vi "GetWSNames.vi"(8 "error in (no error)":errorcluster, 11 "Config":T1) -> (0 "error out":errorcluster, 3 "Names":string[](array[string]))   [LabVIEW 2020]
uses:
  <vilib>/WebServerConfig/Config.ctl
  <vilib>/WebServerConfig/Server.ctl
  <vilib>/WebServerConfig/Alias.ctl
  <vilib>/WebServerConfig/ErrorDocument.ctl
  <vilib>/WebServerConfig/Action.ctl
  <vilib>/WebServerConfig/Redirect.ctl
  <vilib>/WebServerConfig/Interface.ctl
  <vilib>/WebServerConfig/AddHandler.ctl
  <vilib>/WebServerConfig/SSL.ctl
  <vilib>/WebServerConfig/CustomLog.ctl
  <vilib>/WebServerConfig/LoadModule.ctl
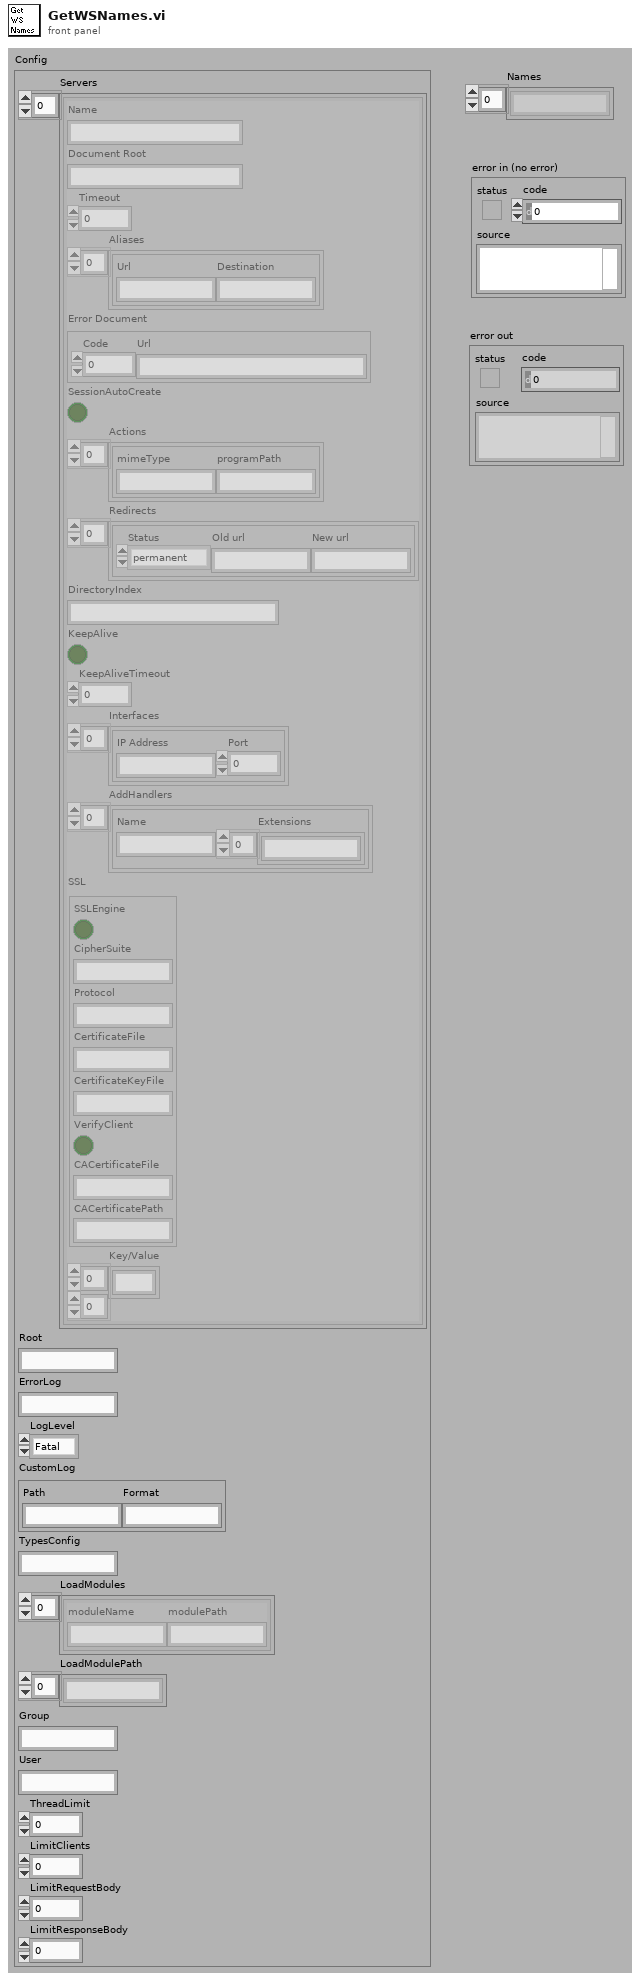
[diagram p1: front panel]
types:
  T1 = typedef "Config.ctl" = cluster{"Servers":T2[], "Root":string, "ErrorLog":string, "LogLevel":enum16{"Fatal", "Error", "Warn", "Info", "Debug", "5", "6", "7", "8", "Verbose"}, "CustomLog":T10, "TypesConfig":string, "LoadModules":T11[], "LoadModulePath":string[], "Group":string, "User":string, "ThreadLimit":u32, "LimitClients":u32, "LimitRequestBody":u32, "LimitResponseBody":u32}
  T2 = typedef "Server.ctl" = cluster{"Name":string, "Document Root":string, "Timeout":u32, "Aliases":T3[], "Error Document":T4, "SessionAutoCreate":bool, "Actions":T5[], "Redirects":T6[], "DirectoryIndex":string, "KeepAlive":bool, "KeepAliveTimeout":u32, "Interfaces":T7[], "AddHandlers":T8[], "SSL":T9, "Key/Value":string[][]}
  T3 = typedef "Alias.ctl" = cluster{"Url":string, "Destination":string}
  T4 = typedef "ErrorDocument.ctl" = cluster{"Code":u16, "Url":string}
  T5 = typedef "Action.ctl" = cluster{"mimeType":string, "programPath":string}
  T6 = typedef "Redirect.ctl" = cluster{"Status":enum16{"permanent", "temp", "seeother", "gone"}, "Old url":string, "New url":string}
  T7 = typedef "Interface.ctl" = cluster{"IP Address":string, "Port":u16}
  T8 = typedef "AddHandler.ctl" = cluster{"Name":string, "Extensions":string[]}
  T9 = typedef "SSL.ctl" = cluster{"SSLEngine":bool, "CipherSuite":string, "Protocol":string, "CertificateFile":string, "CertificateKeyFile":string, "VerifyClient":bool, "CACertificateFile":string, "CACertificatePath":string}
  T10 = typedef "CustomLog.ctl" = cluster{"Path":string, "Format":string}
  T11 = typedef "LoadModule.ctl" = cluster{"moduleName":string, "modulePath":string}
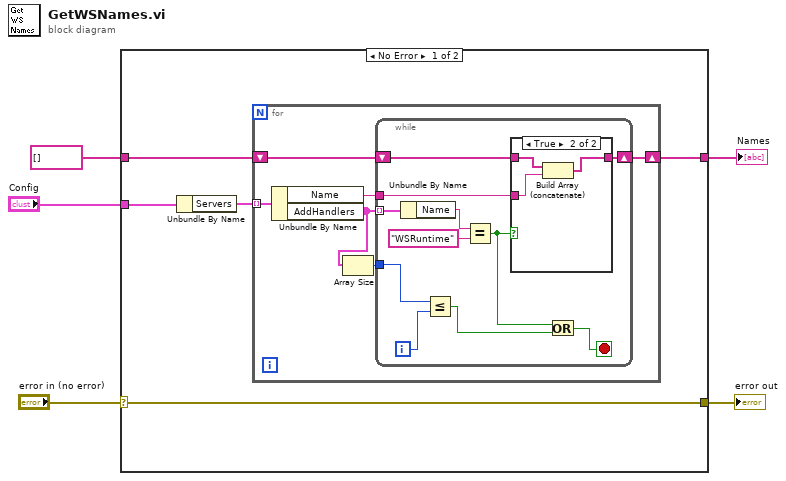
[diagram p0: block diagram]
diagram:
  n1 = case shown="No Error" "error in (no error)" {
    selector: "error in (no error)" -> [w7 w33]
    tunnel: [w9 w32] -> w5
    tunnel: "Config" -> [w8 _]
    tunnel: [w7 w33] -> w2
    tunnel: string[] [] -> [w6 w32]
    frame No Error {
      n2 = Unbundle By Name(w8) -> ("Servers"=w10:T2[])
      n3 = for {
        tunnel: w10 -> [w16] mode=indexing
        shift-right: [w12] -> w9
        shift-left: w6 -> [w11]
        n4 = Unbundle By Name(w16) -> ("Name"=w15:string, "AddHandlers"=w14:T8[])
        n5 = Array Size(array=w14) -> (size(s)=w13:i32)
        n6 = while {
          tunnel: w14 -> [w27] mode=indexing
          tunnel: w15 -> [w19]
          tunnel: w13 -> [w25]
          shift-right: [w18] -> w12
          shift-left: w11 -> [w17]
          i -> [w26]
          stop <- w24 stop-if-true
          n7 = Unbundle By Name(w27) -> ("Name"=w22:string)
          n8 = Less Or Equal?(x=w25, y=w26) -> (x <= y?=w23:bool)
          n9 = Equal?(x=w22, y="WSRuntime") -> (x = y?=w20:bool)
          n10 = case shown="True" w20 {
            tunnel: w19 -> [_ w31]
            tunnel: [w28 w30] -> w18
            tunnel: w17 -> [w28 w29]
            frame False {
            }
            frame True {
              n11 = Build Array (concatenate)(w29, w31) -> (w30:string[])
            }
          }
          n12 = Or(x=w20, y=w23) -> (x .or. y?=w24:bool)
        }
      }
    }
    frame Error {
    }
  }
  "Names" <- w5
  "error out" <- w2
